vi "FG GPS Trail.vi"(2 "FG Action (Read)":T2, 3 "GPS Buffer in":T1 {"Longitude" format="%#_14g"; "Latitude" format="%#_14g"}) -> (1 "GPS Buffer out":T1 {"Longitude" format="%#_14g"; "Latitude" format="%#_14g"})   [LabVIEW 2009]
uses:
  TypeDefs/Sensor TypeDefs/GPS Data.ctl
  Actions for FG's.ctl
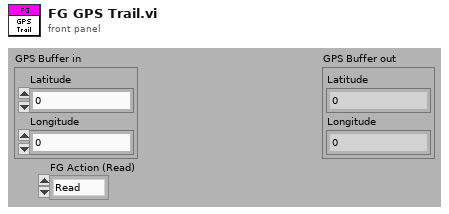
[diagram p1: front panel]
types:
  T1 = typedef "GPS Data.ctl" = cluster{"Latitude":dbl, "Longitude":dbl}
  T2 = typedef "Actions for FG's.ctl" = enum16{"Read", "Write"}
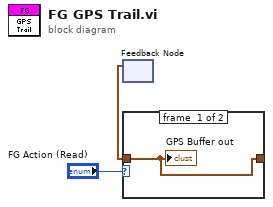
[diagram p0: block diagram]
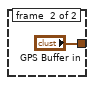
[diagram p2: hidden frame]
diagram:
  n1 = feedback #1() -> (w1:T1)  [unwired: 1 in]
  n2 = case shown="\"Read\", Default" "FG Action (Read)" {
    tunnel: w1 -> [w4 _]
    tunnel: [w4 "GPS Buffer in"] -> w2
    frame #0 {
      "GPS Buffer out" <- w4
    }
    frame #1 {
    }
  }
